vi "UsingChartsAndGraphs.vi"() -> ()   [LabVIEW 2018]
panel:
  out "Waveform Graph":dbl[](graph)
  out "Temperature Value (C)":dbl
  in  "stop":bool
  out "Waveform Chart":dbl(graph)
  in  "Temperature":dbl(slide) scale=0.0..200.0
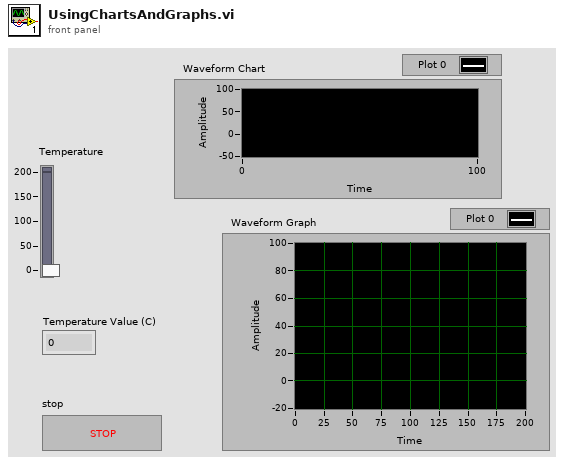
[diagram p1: front panel]
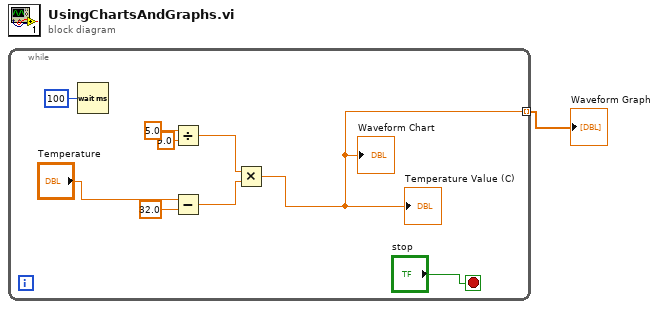
[diagram p0: block diagram]
diagram:
  n1 = while {
    tunnel: [w2] -> w1 mode=indexing
    stop <- "stop" stop-if-true
    n2 = Wait (ms)(milliseconds to wait=u32 100) -> ()  [unwired: 1 out]
    n3 = Divide(x=5.0, y=9.0) -> (x/y=w5:dbl)
    n4 = Subtract(x="Temperature", y=32.0) -> (x-y=w4:dbl)
    n5 = Multiply(x=w5, y=w4) -> (x*y=w2:dbl)
    "Waveform Chart" <- w2
    "Temperature Value (C)" <- w2
  }
  "Waveform Graph" <- w1
